vi "CAN_parse_BMS_2_temp.vi"(11 "CAN message data 2":u8[](array[numeric])) -> ()   [LabVIEW 2018]
uses:
  Type_Def/TypeDef_BMSDatas.ctl
  Type_Def/TypeDef_BMSStatuss.ctl
  <vilib>/CANopenLib/CANOPEN.llb/CANopen Fetch from Data [U16].vi
panel:
  out "output cluster":T1
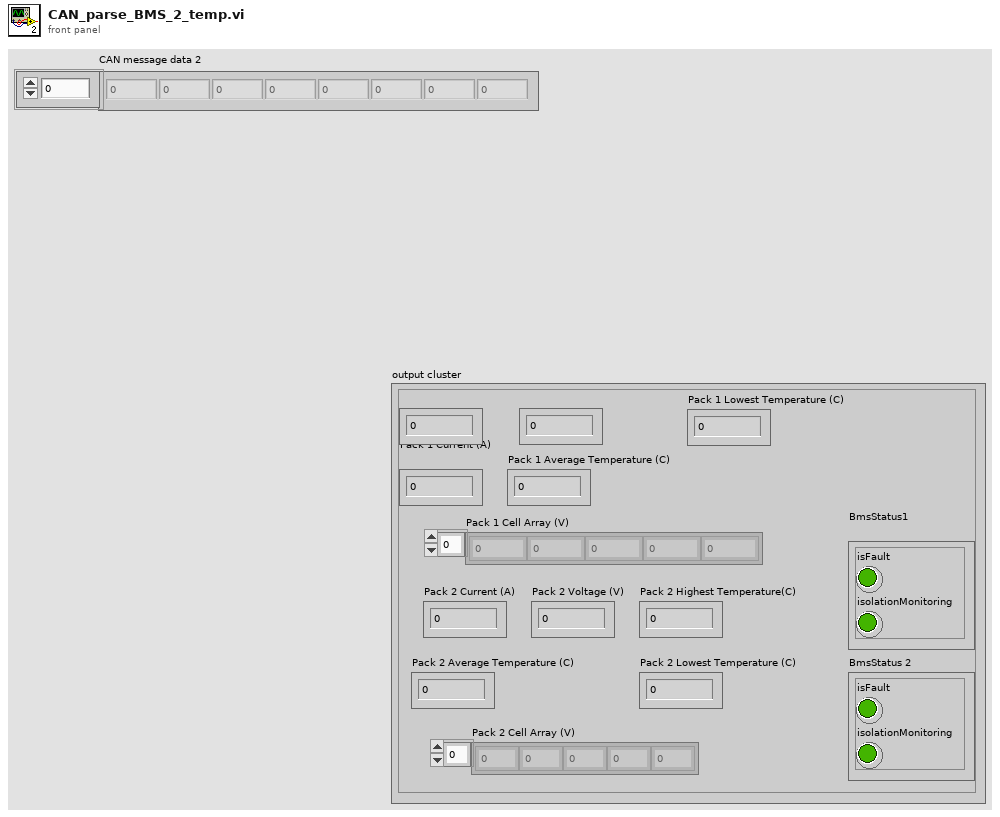
[diagram p1: front panel]
types:
  T1 = typedef "TypeDef_BMSDatas.ctl" = cluster{"Pack 1 Current (A)":dbl, "Pack 1 Voltage (V)":dbl, "Pack 1 Highest Temperature(C)":dbl, "BmsStatus1":T2, "Pack 2 Current (A)":dbl, "Pack 2 Voltage (V) ":dbl, "Pack 2 Highest Temperature(C) ":dbl, "BmsStatus 2":T2, "Pack 1 Cell Array (V)":dbl[], "Pack 2 Cell Array (V)":dbl[], "Pack 1 Lowest Temperature (C)":dbl, "Pack 1 Average Temperature (C)":dbl, "Pack 2 Average Temperature (C)":dbl, "Pack 2 Lowest Temperature (C)":dbl}
  T2 = typedef "TypeDef_BMSStatuss.ctl" = cluster{"isFault":bool, "isolationMonitoring":bool}
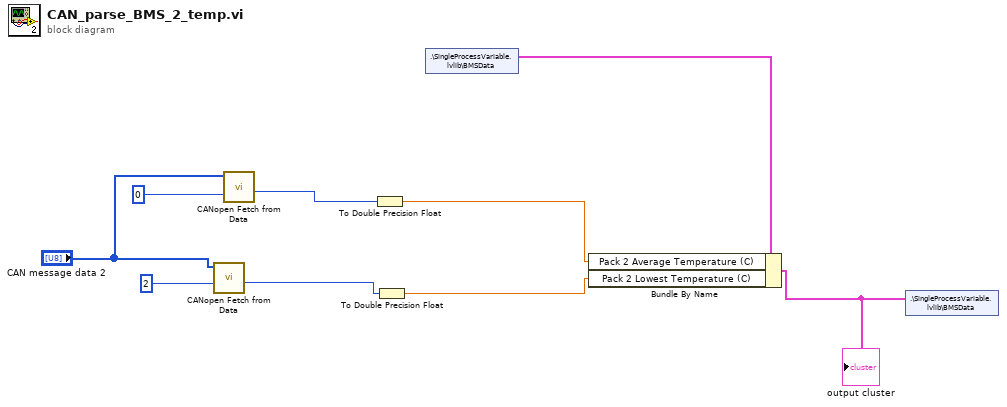
[diagram p0: block diagram]
diagram:
  n1 = call-poly <vilib>:"CANopen Fetch from Data.vi"("offset (0)"=2, "CANopen data in"="CAN message data 2") -> ("unsigned 16-bit integer"=w4:u16)  [unwired: 7 in, 2 out]
  n2 = call-poly <vilib>:"CANopen Fetch from Data.vi"("offset (0)"=0, "CANopen data in"="CAN message data 2") -> ("unsigned 16-bit integer"=w7:u16)  [unwired: 7 in, 2 out]
  n3 = To Double Precision Float(number=w7) -> (double precision float=w2:dbl)
  n4 = To Double Precision Float(number=w4) -> (double precision float=w1:dbl)
  n5 = shared-variable ".\\SingleProcessVariable.lvlib\\BMSData"() -> (w9:T1)  [unwired: 1 in, 1 out]
  n6 = Bundle By Name(cluster=w9, "Pack 2 Average Temperature (C)"=w2, "Pack 2 Lowest Temperature (C)"=w1) -> (w8:T1)
  "output cluster" <- w8
  n7 = shared-variable ".\\SingleProcessVariable.lvlib\\BMSData"(w8) -> ()  [unwired: 1 in, 1 out]
